vi "connect.vi"(6 "timeout (25000ms)":i32=25000, 8 "error in (no error)":errorcluster, 9 "Target":T1="DDM", 10 "physical connection":string, 11 "daemon reference in":refnum<k5>) -> (0 "error out":errorcluster, 2 "response":string, 3 "daemon reference out":refnum<k5>, 4 "parameter(s) out":string, 5 "command out":string="connect")   [LabVIEW 2017]
doc: "<b>Command: </b>\"connect\"\n\n<b>Description: </b> This command connects the Daemon to a physical BUS connection. This command must be called to establish a connection to the DIPC device after which other DIPC based commands can be ran.\n\n<b>Parameters: </b>\n\n 1. Address (Serial port [COM] or network address [IP:PORT])\n____________________________________________\nDIPC 692 Daemon API 10.0.0.1\nSam Tee - Dyson Technology Ltd\nCopyright (c) 2024, Dyson Technology Ltd"
uses:
  typdef/destination.ctl
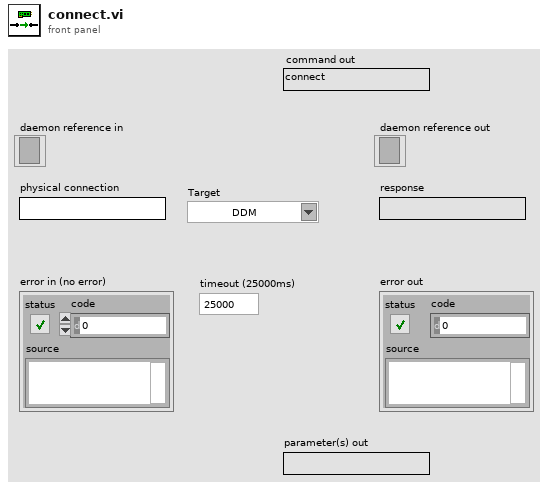
[diagram p1: front panel]
types:
  T1 = typedef "destination.ctl" = string
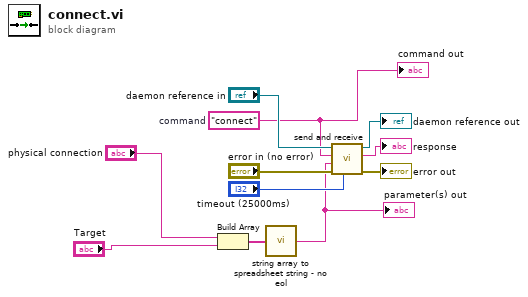
[diagram p0: block diagram]
diagram:
  w9 = "connect"  # command
  n1 = Build Array("physical connection", "Target") -> (w3:T1[])
  n2 = call "string array to spreadsheet string - no eol.vi"("string array"=w3) -> ("spreadsheet string - no eol"=w2:string)
  "parameter(s) out" <- w2
  n3 = call "send and receive.vi"("timeout (25000ms)"="timeout (25000ms)", "error in (no error)"="error in (no error)", "data"=w2, "command"=w9, "daemon reference in"="daemon reference in") -> ("error out"=→"error out":errorcluster, "response"=→"response":string, "daemon reference out"=→"daemon reference out":refnum<k5>)  [unwired: 4 in]
  "command out" <- w9
